vi "Lead Screw Control.vi"() -> ()   [LabVIEW 2012]
uses:
  Robot Global Data.vi
panel:
  out "front":bool
  out "rear":bool
  out "x-y":dbl
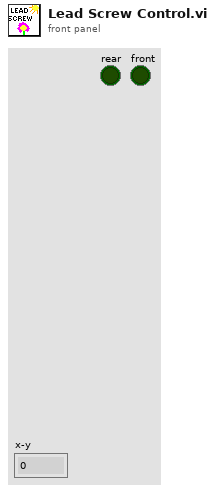
[diagram p1: front panel]
types:
  T1 = typedef "WPI_MotorControlDeviceRef.ctl" = cluster{"DeviceStatus":errorcluster, "Type":enum16{"PWM", "CAN"}, "PWM":cluster{"Digital Module":T2, "PWM Channel":T3, "DeadBand":T4}, "CAN":cluster{"Device Number":u8, "Control Mode":T5, "Semaphore":T6, "Max Vout":dbl}, "Invert":bool, "TransformRef":T7, "InvTransformRef":T7}
  T2 = typedef "FPGA_TypedefDigitalModule.ctl" = enum16{"Digital Module 1", "Digital Module 2"}
  T3 = typedef "FPGA_DIOPWMChannel.ctl" = enum8{"PWM 1", "PWM 2", "PWM 3", "PWM 4", "PWM 5", "PWM 6", "PWM 7", "PWM 8", "PWM 9", "PWM 10", "Invalid"}
  T4 = typedef "WPI_PWMDeadband.ctl" = cluster{"Name":string, "maxPositivePwm":i32, "minPositivePwm":i32, "centerPwm":i32, "maxNegativePwm":i32, "minNegativePwm":i32, "angularRange":u16}
  T5 = typedef "WPI_CANJaguar_ControlMode.ctl" = enum8{"Percent VBus", "Current", "Speed", "Position", "Voltage"}
  T6 = typedef "Semaphore RefNum" = refnum<k1>
  T7 = typedef "WPI_PWMTransform_ConPane.ctl" = refnum<vi>
  T8 = typedef "WPI_DigitalInputDevRef.ctl" = cluster{"DevStatus":errorcluster, "DIO Channel":T9, "Digital Module":T2}
  T9 = typedef "FPGA_DIOChannel.ctl" = enum8{"DIO 1", "DIO 2", "DIO 3", "DIO 4", "DIO 5", "DIO 6", "DIO 7", "DIO 8", "DIO 9", "DIO 10", "DIO 11", "DIO 12", "DIO 13", "DIO 14", "Invalid"}
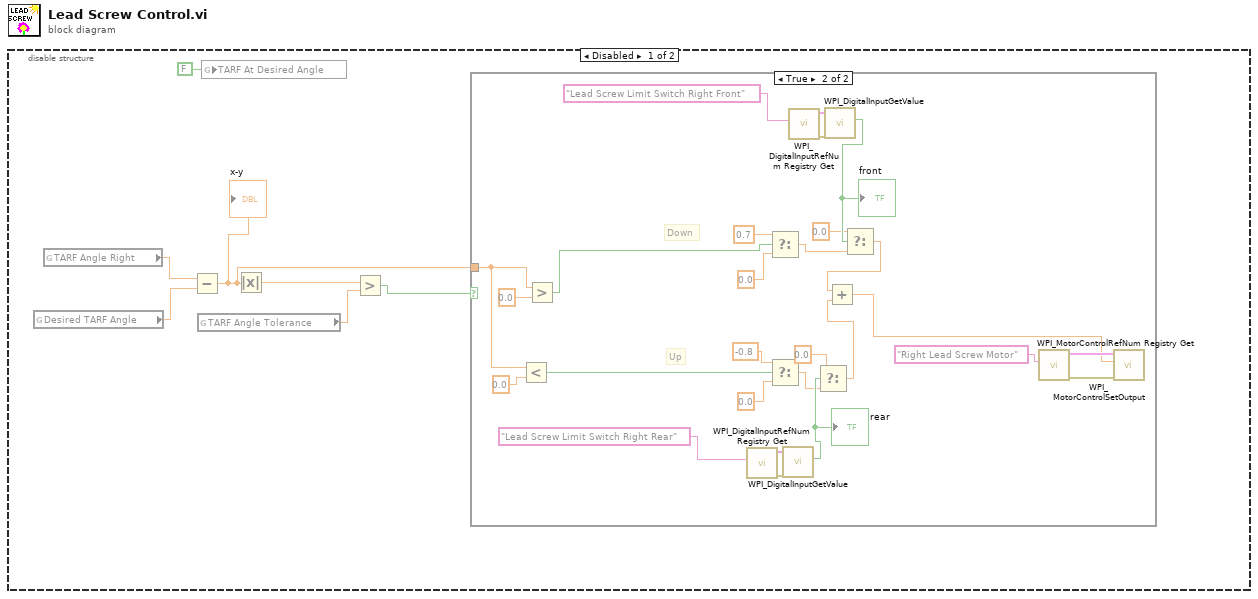
[diagram p0: block diagram]
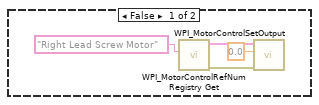
[diagram p2: hidden frame]
diagram:
  n1 = disable-structure shown="Disabled" {
    frame Disabled {
      n2 = global read "Robot Global Data.vi" "Desired TARF Angle"() -> (w4:dbl)
      n3 = global read "Robot Global Data.vi" "TARF Angle Right"() -> (w5:dbl)
      n4 = Subtract(x=w5, y=w4) -> (x-y=w1:dbl)
      "x-y" <- w1
      n5 = global read "Robot Global Data.vi" "TARF Angle Tolerance"() -> (w6:dbl)
      n6 = global write "Robot Global Data.vi" "TARF At Desired Angle"(FALSE ("TARF At Desired Angle")) -> ()
      n7 = Absolute Value(x=w1) -> (abs(x)=w7:dbl)
      n8 = Greater?(x=w7, y=w6) -> (0:w2:bool)
      n9 = case shown="True" w2 {
        tunnel: w1 -> [_ w13]
        frame False {
          n10 = call <vilib>:"WPI_MotorControlRefNum Registry Get.vi"("refnum name"="Right Lead Screw Motor") -> ("error out"=w9:errorcluster, "MotorControlDevRef"=w10:T1)  [unwired: 9 in]
          n11 = call <vilib>:"WPI_MotorControlSetOutput.vi"("error in (no error)"=w9, "Output"=0.0, "MotorControlDevRef"=w10) -> ()  [unwired: 6 in, 3 out]
        }
        frame True {
          # "Up"
          # "Down"
          n12 = Less?(x=w13, y=0.0) -> (x < y?=w14:bool)
          n13 = Greater?(x=w13, y=0.0) -> (0:w15:bool)
          n14 = call <vilib>:"WPI_DigitalInputRefNum Registry Get.vi"("refnum name"="Lead Screw Limit Switch Right Rear") -> ("error out"=w24:errorcluster, "DigitalInputDevRef"=w23:T8)  [unwired: 9 in]
          n15 = Select(t=0.7, s=w15, f=0.0) -> (s? t:f=w20:dbl)
          n16 = Select(t=-0.8, s=w14, f=0.0) -> (s? t:f=w18:dbl)
          n17 = call <vilib>:"WPI_DigitalInputGetValue.vi"("error in (no error)"=w24, "DigitalInputDevRef"=w23) -> ("Value"=w21:bool)  [unwired: 7 in, 2 out]
          "rear" <- w21
          n18 = call <vilib>:"WPI_DigitalInputRefNum Registry Get.vi"("refnum name"="Lead Screw Limit Switch Right Front") -> ("error out"=w28:errorcluster, "DigitalInputDevRef"=w27:T8)  [unwired: 9 in]
          n19 = Select(t=0.0 ("f"), s=w21, f=w18) -> (s? t:f=w30:dbl)
          n20 = call <vilib>:"WPI_DigitalInputGetValue.vi"("error in (no error)"=w28, "DigitalInputDevRef"=w27) -> ("Value"=w26:bool)  [unwired: 7 in, 2 out]
          "front" <- w26
          n21 = Select(t=0.0, s=w26, f=w20) -> (s? t:f=w29:dbl)
          n22 = Add(x=w29, y=w30) -> (x+y=w35:dbl)
          n23 = call <vilib>:"WPI_MotorControlRefNum Registry Get.vi"("refnum name"="Right Lead Screw Motor") -> ("error out"=w36:errorcluster, "MotorControlDevRef"=w37:T1)  [unwired: 9 in]
          n24 = call <vilib>:"WPI_MotorControlSetOutput.vi"("error in (no error)"=w36, "Output"=w35, "MotorControlDevRef"=w37) -> ()  [unwired: 6 in, 3 out]
        }
      }
    }
    frame Enabled {
    }
  }
